vi "Write Index.vi"(8 "error in (no error)":errorcluster, 10 "Index":i32, 11 "Elf in":refnum<class "Elf.lvclass">) -> (0 "error out":errorcluster, 3 "Elf out":refnum<class "Elf.lvclass">)   [LabVIEW 2017, in "Elf.lvclass"]
uses:
  Elf.lvclass
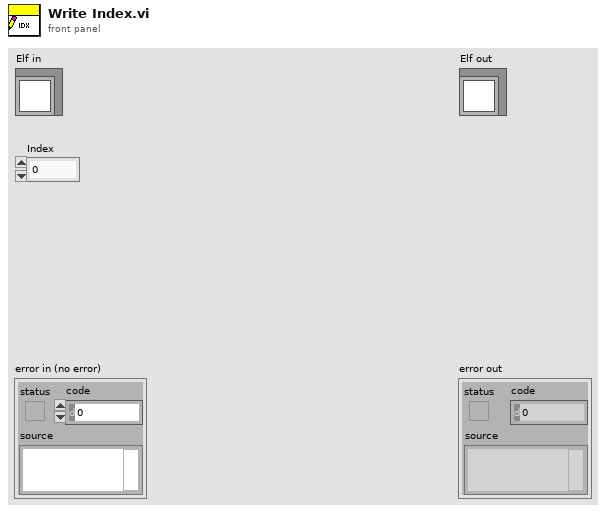
[diagram p1: front panel]
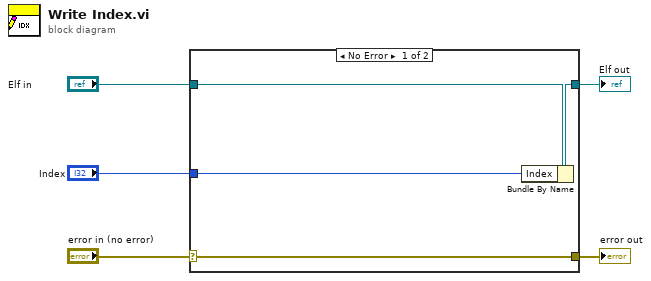
[diagram p0: block diagram]
diagram:
  n1 = case shown="No Error" "error in (no error)" {
    selector: "error in (no error)" -> [w9 w10]
    tunnel: [w9 w10] -> w4
    tunnel: [w7 w11] -> w2
    tunnel: "Elf in" -> [w8 w11]
    tunnel: "Index" -> [w6 _]
    frame No Error {
      n2 = Bundle By Name(cluster=w8, "Index"=w6) -> (w7:refnum<class "Elf.lvclass">)
    }
    frame Error {
    }
  }
  "error out" <- w4
  "Elf out" <- w2
